vi "Configure CALC1 Math Calculation.vi"(8 "error in (no error)":errorcluster, 9 "Enable CALC 1 Calculation (T: Enable)":bool=TRUE, 10 "Calculation Format (2: Polynomial)":i32(ring)=2 items=["NONE", "Percent", "Polynomial", "Ratio", "Deviation", "Percent deviation", "Logarithmic base 10", "Linear"], 11 "VISA resource name":refnum<visa-resource-name>) -> (0 "error out":errorcluster, 3 "VISA resource name out":refnum<visa-resource-name>)   [LabVIEW 2016, in "Keithley 6517.lvlib"]
doc: "Enables or disables the CALC 1 calculation and configures the format for the CALC 1 math calculation.\n\n<B>Note:</B>\nFor model <B>6514</B>, control <B>Calculation Format</B> can only be set to <B>Percent</B> and <B>Linear</B>."
uses:
  <instrlib>/Keithley 6517/Keithley 6517.lvlib
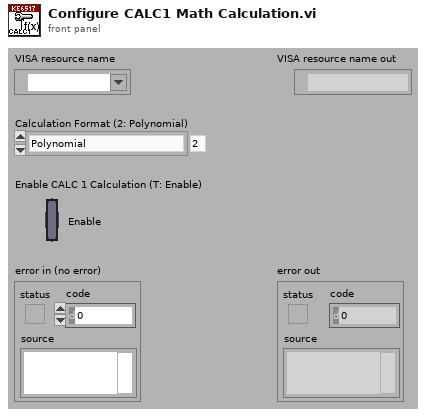
[diagram p1: front panel]
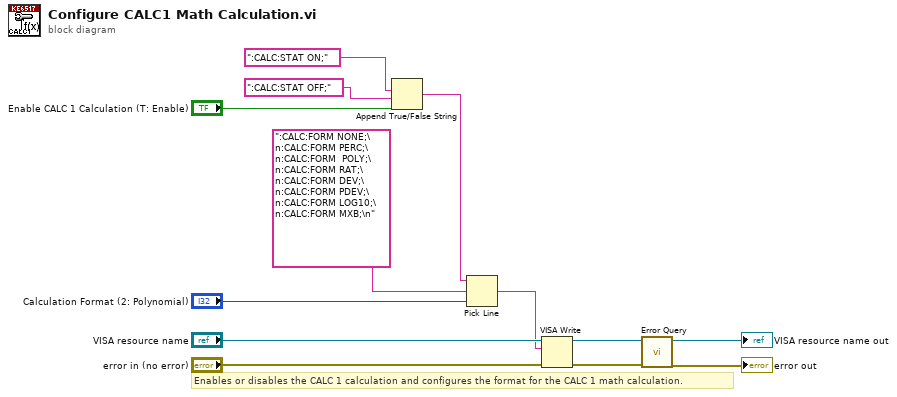
[diagram p0: block diagram]
diagram:
  # "Enables or disables the CALC 1 calculation and configures the format for the CALC 1 math calculation."
  n1 = Append True/False String(1:"Enable CALC 1 Calculation (T: Enable)", 2:":CALC:STAT OFF;", 3:":CALC:STAT ON;") -> (0:w1:string)  [unwired: 1 in]
  n2 = Pick Line(string ("")=w1, multi-line string=":CALC:FORM NONE;\n:CALC:FORM PERC;\n:CALC:FORM  POLY;\n:CALC:FORM RAT;\n:CALC:FORM DEV;\n:CALC:FORM PDEV;\n:CALC:FORM LOG10;\n:CALC:FORM MXB;\n", line index="Calculation Format (2: Polynomial)") -> (output string=w2:string)
  n3 = VISA Write(VISA resource name="VISA resource name", write buffer=w2, error in (no error)="error in (no error)") -> (VISA resource name out=w8:refnum<visa-resource-name>, error out=w7:errorcluster)  [unwired: 1 out]
  n4 = call <instrlib>:"Error Query.vi"("error in (no error)"=w7, "VISA resource name"=w8) -> ("error out"=→"error out":errorcluster, "VISA resource name out"=→"VISA resource name out":refnum<visa-resource-name>)  [unwired: 6 in, 2 out]
